vi "Receive Ack.vi"(8 "error in (no error)":errorcluster, 11 "RemoteControl.ZMQ in":refnum<class "RemoteControl.ZMQ.lvclass">) -> (0 "error out":errorcluster, 2 "Command Sent":string, 3 "RemoteControl.ZMQ out":refnum<class "RemoteControl.ZMQ.lvclass">)   [LabVIEW 2019, in "RemoteControl.ZMQ.lvclass"]
uses:
  RemoteControl.ZMQ.lvclass
  <vilib>/addons/zeromq/zmq_socket.lvclass
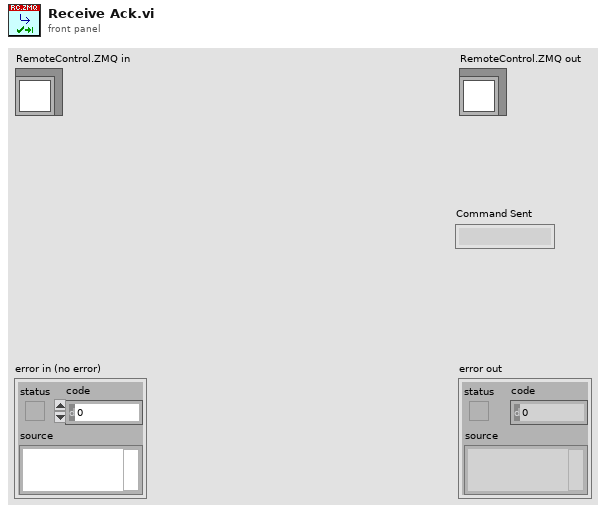
[diagram p1: front panel]
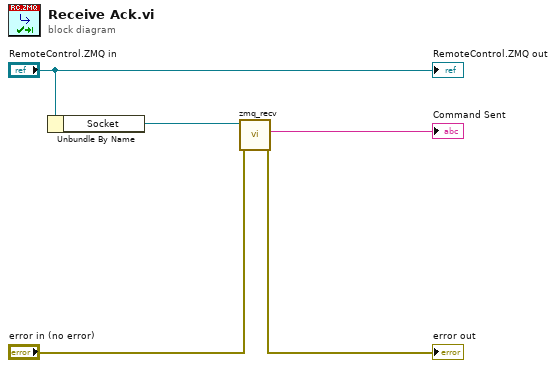
[diagram p0: block diagram]
diagram:
  n1 = Unbundle By Name("RemoteControl.ZMQ in") -> ("Socket"=w3:refnum<class "zmq_socket.lvclass">)
  n2 = call <vilib>:"zmq_recv.vi"("error in"="error in (no error)", "socket in"=w3) -> ("error out"=→"error out":errorcluster, "data"=→"Command Sent":string)  [unwired: 3 in, 3 out]
  "RemoteControl.ZMQ out" <- "RemoteControl.ZMQ in"
